vi "niRFUtil CONV Real WDT to Real Waveform.vi"(7 "Real WDT":T1) -> (8 "Real Waveform":T2 {"y" min=0 max=127 format="%.2f"; "dx" format="%^.2e"; "x0" format="%^.2e"})   [LabVIEW 2015, in "niRFUtil.lvlib"]
uses:
  niRFUtil.lvlib
  Includes/niRFUtil INC Real Waveform.ctl
  Includes/niRFUtil INC Real Array.ctl
  Includes/niRFUtil INC Real WDT.ctl
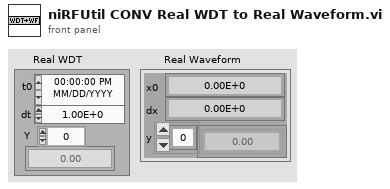
[diagram p1: front panel]
types:
  T1 = typedef "niRFUtil.lvlib/niRFUtil INC Real WDT.ctl" = waveform(sgl)
  T2 = typedef "niRFUtil.lvlib/niRFUtil INC Real Waveform.ctl" = cluster{"x0":dbl, "dx":dbl, "y":T3}
  T3 = typedef "niRFUtil.lvlib/niRFUtil INC Real Array.ctl" = sgl[]
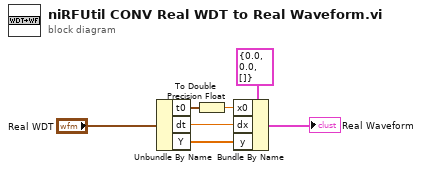
[diagram p0: block diagram]
diagram:
  n1 = Unbundle By Name("Real WDT") -> ("t0"=w4:timestamp, "dt"=w6:dbl, "Y"=w5:sgl[])
  n2 = To Double Precision Float(number=w4) -> (double precision float=w3:dbl)
  n3 = Bundle By Name(cluster=T2 {"x0"=0.0, "dx"=0.0, "y"=[]} ("Real Waveform"), "x0"=w3, "dx"=w6, "y"=w5) -> (→"Real Waveform":T2)
